vi "Create and Read CDO.vi"(8 "error in":errorcluster, 9 "drive from slot in":T1, 10 "channel settings in":T2[](array[typedef]), 11 "Module Test in":refnum<class "Module Test.lvclass">) -> (0 "error out":errorcluster, 1 "drive from slot out":T1, 2 "channel settings out":T2[](array[typedef]), 3 "Module Test out":refnum<class "Module Test.lvclass">)   [LabVIEW 2019, in "Module Test.lvclass"]
uses:
  Module Test.lvclass
  Scripting/Modules/Mode Classes/Controls/counter driven output channel settings.ctl
  Scripting/Modules/Channel Classes/Counter Driven Output Channel/Counter Driven State.ctl
  Scripting/Modules/Mode Classes/Counter Driven Output Mode/Drive from Slot.ctl
  Scripting/Modules/Channel Classes/Counter Driven Output Channel/Counter Driven Output Channel.lvclass
  Scripting/Scan Engine Scripting.lvlib
  Scripting/Modules/Mode Classes/Counter Driven Output Mode/Counter Driven Output Mode.lvclass
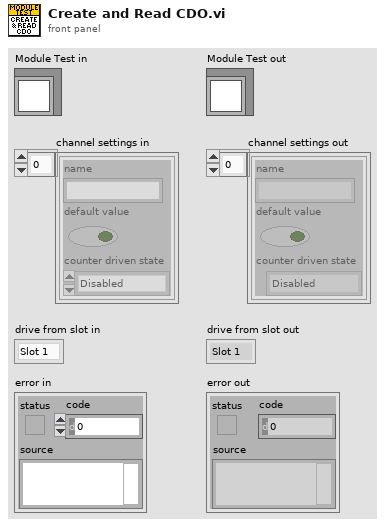
[diagram p1: front panel]
types:
  T1 = typedef "Scan Engine Scripting.lvlib/Counter Driven Output Mode.lvclass/Drive from Slot.ctl" = enum16{"Slot 1", "Slot 2", "Slot 3", "Slot 4", "Slot 5", "Slot 6", "Slot 7", "Slot 8"}
  T2 = typedef "Scan Engine Scripting.lvlib/counter driven output channel settings.ctl" = cluster{"name":string, "default value":bool, "counter driven state":T3}
  T3 = typedef "Scan Engine Scripting.lvlib/Counter Driven Output Channel.lvclass/Counter Driven State.ctl" = enum16{"Disabled", "Enabled"}
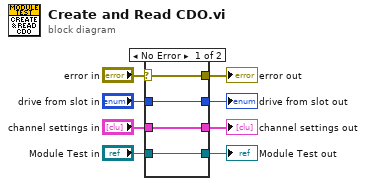
[diagram p0: block diagram]
diagram:
  n1 = case shown="No Error" "error in" {
    selector: "error in" -> [w11 w16]
    tunnel: [w11 w16] -> w7
    tunnel: [w12 w15] -> w5
    tunnel: "Module Test in" -> [w12 w15]
    tunnel: "channel settings in" -> [w10 w14]
    tunnel: [w10 w14] -> w3
    tunnel: "drive from slot in" -> [w9 w13]
    tunnel: [w9 w13] -> w1
    frame No Error {
    }
    frame Error {
    }
  }
  "error out" <- w7
  "Module Test out" <- w5
  "channel settings out" <- w3
  "drive from slot out" <- w1
